vi "Test2_3a_ASIC_mezzanineNEW.vi"(4 "Voltages comprobation":dbl[](array[numeric])=[0.05, 0.1, 0.2, 0.3, 0.4, 0.5, 0.6, 0.7, 0.8, 1.0], 6 "IB_Clip":i32[](array[numeric])=[7, 15, 23, 31, 39, 47, 55, 63], 7 "Report Enable":bool, 8 "error in":errorcluster, 9 "Cycles Burst":i32=10000, 10 "Channels":i32[](array[numeric])=[0, 1, 2, 3, 4, 5, 6], 11 "Instrument VISA in":T1={"AWG VISA"="generadorpulsos", "Oscilloscope  VISA "="Oscilloscope", "Integration Board IP"="172.16.7.43", "connection ID"=refnum, "report out"=refnum, "report file path"=path "D:/CTA/Data_test/ASIC/chip_test"}) -> (0 "error out":errorcluster, 3 "Instrument VISA out":T1={"AWG VISA"="generadorpulsos", "Oscilloscope  VISA "="Oscilloscope", "Integration Board IP"="172.16.7.43", "connection ID"=refnum, "report out"=refnum, "report file path"=path "D:/CTA/Data_test/test3a"})   [LabVIEW 2009]
uses:
  <vilib>/Utility/NIReport.llb/NI_report.lvclass
  <vilib>/Utility/NIReport.llb/HTML/NI_HTML.lvclass
  <instrlib>/Agilent 8000 Series/Public/Configure/Configure Math (Binary Operation).vi
  <instrlib>/Agilent 8000 Series/Public/Data/Read (Multiple Waveforms).vi
  <instrlib>/Agilent 81150/Agilent 81150.lvlib
  L0_Asic/L0 Asic Test Folder v9/C/Program Files/National Instruments/LabVIEW 2012/instr.lib/Agilent 8000 Series/Agilent 8000 Series.lvlib
panel:
  in  "Selected Delay":i32=1
  in  "Atenuation":i32[](array[numeric])=[0, 4, 8, 12]
  in  "Generador enable?":bool=TRUE
  out "dt":dbl
  out "report file path":path=path "D:/CTA/Data_test/ASIC/chip_test"
  in  "Full waveform":bool
  out "Waveform Data":waveform(dbl)[](graph)
  out "x-y 4":u32=4294966934
  in  "y":dbl=250.0
  out "bucle":u16=32
  out "x-y 3":u32
  out "points quantity":dbl=10.0
  out "appended array":dbl[](array[numeric])=[9.99999e+37, 9.99999e+37, 9.99999e+37, 9.99999e+37, 0.028568, 0.000458, 2.716396e-09, 8.8051e-11, 1.4000634e-08, 8.5636e-11, 10.0]
  out "read buffer 3":string="V amptd(1),9.99999E+37,9.99999E+37,9.99999E+37,9.99999E+37,9.99999E+37,1.0E+01,+ width(1),9.99999E+37,9.99999E+37,9.99999E+37,9.99999E+37,9.99999E+37,9.99999E+37,V amptd(f2),2.861E-02,2.776E-02,2.904E-02,2.8568E-02,4.58E-04,1.0E+01,+ width(f2),2.81643E-09,2.57734E-09,2.81643E-09,2.716396E-09,8.8051E-11,1.0E+01,Time(1-f2),1.406011E-08,1.390256E-08,1.414073E-08,1.4000634E-08,8.5636E-11,1.0E+01\n"
  out "x-y":u32=372
  out "Numeric":i32=179238008
  in  "Att gain":u32=4095
  in  "Save NOW!":bool
  in  "End 2":bool
  out "Data output":dbl[][](array[numeric])=[[0.05, 0.0, 0.0, 0.0, 1.0, 9.99999e+37, 9.99999e+37, 9.99999e+37, 9.99999e+37, 9.99999e+37, 9.99999e+37, 9.99999e+37, 9.99999e+37, 9.99999e+37, 9.99999e+37, 11.0, 0.0336, 0.007807142857142857, 0.0], [0.05, 0.0, 0.0, 1.0, 1.0, 9.99999e+37, 9.99999e+37, 9.99999e+37, 9.99999e+37, 0.02322, 0.00108, 2.92182e-09, 1.2099e-10, 1.426508e-08, 1.0426e-10, 9.0, 0.0336, 0.007807142857142857, 1.0], [0.05, 0.0, 0.0, 2.0, 1.0, 9.99999e+37, 9.99999e+37, 9.99999e+37, 9.99999e+37, 0.027616, 0.00075, 2.762328e-09, 1.20518e-10, 1.396173e-08, 9.0461e-11, 10.0, 0.0336, 0.007807142857142857, 2.0], [0.05, 0.0, 0.0, 3.0, 1.0, 9.99999e+37, 9.99999e+37, 9.99999e+37, 9.99999e+37, 0.029619, 0.000653, 2.613329e-09, 9.9889e-11, 1.3763225e-08, 1.01914e-10, 10.0, 0.0336, 0.007807142857142857, 3.0], [0.05, 0.0, 0.0, 4.0, 1.0, 9.99999e+37, 9.99999e+37, 9.99999e+37, 9.99999e+37, 0.030934, 0.001529, 2.609376e-09, 5.0257e-11, 1.370877e-08, 6.3168e-11, 10.0, 0.0336, 0.007807142857142857, 4.0], [0.05, 0.0, 0.0, 5.0, 1.0, 9.99999e+37, 9.99999e+37, 9.99999e+37, 9.99999e+37, 0.031684, 0.000984, 2.569953e-09, 8.8766e-11, 1.3621526e-08, 6.259e-11, 10.0, 0.0336, 0.007807142857142857, 5.0], [0.05, 0.0, 0.0, 6.0, 1.0, 9.99999e+37, 9.99999e+37, 9.99999e+37, 9.99999e+37, 0.031778, 0.000782, 2.551811e-09, 9.6553e-11, 1.3593361e-08, 7.619e-11, 11.0, 0.0336, 0.007807142857142857, 6.0], [0.05, 1.0, 0.0, 0.0, 1.0, 9.99999e+37, 9.99999e+37, 9.99999e+37, 9.99999e+37, 9.99999e+37, 9.99999e+37, 9.99999e+37, 9.99999e+37, 1.011019e-08, 9.9856e-10, 10.0, 0.0336, 0.007807142857142857, 7.0], [0.05, 1.0, 0.0, 1.0, 1.0, 9.99999e+37, 9.99999e+37, 9.99999e+37, 9.99999e+37, 0.02143, 0.001274, 3.059757e-09, 1.55908e-10, 1.4327756e-08, 8.9144e-11, 10.0, 0.0336, 0.007807142857142857, 8.0], [0.05, 1.0, 0.0, 2.0, 1.0, 9.99999e+37, 9.99999e+37, 9.99999e+37, 9.99999e+37, 0.026315, 0.000821, 2.807153e-09, 5.1637e-11, 1.396698e-08, 1.01676e-10, 10.0, 0.0336, 0.007807142857142857, 9.0], [0.05, 1.0, 0.0, 3.0, 1.0, 9.99999e+37, 9.99999e+37, 9.99999e+37, 9.99999e+37, 0.028856, 0.001014, 2.729925e-09, 8.219e-11, 1.3780327e-08, 8.7828e-11, 10.0, 0.0336, 0.007807142857142857, 10.0], [0.05, 1.0, 0.0, 4.0, 1.0, 9.99999e+37, 9.99999e+37, 9.99999e+37, 9.99999e+37, 0.029136, 0.001454, 2.665592e-09, 8.3971e-11, 1.3697819e-08, 7.5969e-11, 10.0, 0.0336, 0.007807142857142857, 11.0], [0.05, 1.0, 0.0, 5.0, 1.0, 9.99999e+37, 9.99999e+37, 9.99999e+37, 9.99999e+37, 0.030325, 0.001136, 2.605316e-09, 7.6693e-11, 1.3613156e-08, 9.0082e-11, 10.0, 0.0336, 0.007807142857142857, 12.0], [0.05, 1.0, 0.0, 6.0, 1.0, 9.99999e+37, 9.99999e+37, 9.99999e+37, 9.99999e+37, 0.030542, 0.000695, 2.600691e-09, 7.2879e-11, 1.3579529e-08, 7.3212e-11, 11.0, 0.0336, 0.007807142857142857, 13.0], [0.05, 2.0, 0.0, 0.0, 1.0, 9.99999e+37, 9.99999e+37, 9.99999e+37, 9.99999e+37, 9.99999e+37, 9.99999e+37, 9.99999e+37, 9.99999e+37, 9.99999e+37, 9.99999e+37, 10.0, 0.0336, 0.007807142857142857, 14.0], [0.05, 2.0, 0.0, 1.0, 1.0, 9.99999e+37, 9.99999e+37, 9.99999e+37, 9.99999e+37, 0.019386, 0.000608, 3.093134e-09, 1.37969e-10, 1.428753e-08, 1.14612e-10, 10.0, 0.0336, 0.007807142857142857, 15.0], [0.05, 2.0, 0.0, 2.0, 1.0, 9.99999e+37, 9.99999e+37, 9.99999e+37, 9.99999e+37, 0.024483, 0.000731, 2.928339e-09, 1.06101e-10, 1.4002377e-08, 6.2052e-11, 10.0, 0.0336, 0.007807142857142857, 16.0], [0.05, 2.0, 0.0, 3.0, 1.0, 9.99999e+37, 9.99999e+37, 9.99999e+37, 9.99999e+37, 0.027198, 0.001369, 2.781238e-09, 5.6434e-11, 1.386892e-08, 9.0615e-11, 11.0, 0.0336, 0.007807142857142857, 17.0], [0.05, 2.0, 0.0, 4.0, 1.0, 9.99999e+37, 9.99999e+37, 9.99999e+37, 9.99999e+37, 0.029441, 0.001219, 2.623158e-09, 6.7678e-11, 1.3704754e-08, 8.6571e-11, 11.0, 0.0336, 0.007807142857142857, 18.0], [0.05, 2.0, 0.0, 5.0, 1.0, 9.99999e+37, 9.99999e+37, 9.99999e+37, 9.99999e+37, 0.030537, 0.000977, 2.611114e-09, 5.8592e-11, 1.365028e-08, 5.1809e-11, 10.0, 0.0336, 0.007807142857142857, 19.0], [0.05, 2.0, 0.0, 6.0, 1.0, 9.99999e+37, 9.99999e+37, 9.99999e+37, 9.99999e+37, 0.031627, 0.000829, 2.563156e-09, 7.6101e-11, 1.3573521e-08, 7.8038e-11, 11.0, 0.0336, 0.007807142857142857, 20.0], [0.05, 3.0, 0.0, 0.0, 1.0, 9.99999e+37, 9.99999e+37, 9.99999e+37, 9.99999e+37, 9.99999e+37, 9.99999e+37, 9.99999e+37, 9.99999e+37, 9.99999e+37, 9.99999e+37, 10.0, 0.0336, 0.007807142857142857, 21.0], [0.05, 3.0, 0.0, 1.0, 1.0, 9.99999e+37, 9.99999e+37, 9.99999e+37, 9.99999e+37, 0.023426, 0.000976, 2.943703e-09, 1.24879e-10, 1.4377233e-08, 6.3364e-11, 10.0, 0.0336, 0.007807142857142857, 22.0], [0.05, 3.0, 0.0, 2.0, 1.0, 9.99999e+37, 9.99999e+37, 9.99999e+37, 9.99999e+37, 0.027462, 0.001241, 2.749469e-09, 8.035e-11, 1.407543e-08, 9.5871e-11, 10.0, 0.0336, 0.007807142857142857, 23.0], [0.05, 3.0, 0.0, 3.0, 1.0, 9.99999e+37, 9.99999e+37, 9.99999e+37, 9.99999e+37, 0.030115, 0.000527, 2.608621e-09, 5.3293e-11, 1.3888327e-08, 4.0853e-11, 10.0, 0.0336, 0.007807142857142857, 24.0], [0.05, 3.0, 0.0, 4.0, 1.0, 9.99999e+37, 9.99999e+37, 9.99999e+37, 9.99999e+37, 0.030314, 0.000803, 2.543724e-09, 8.472e-11, 1.3780628e-08, 6.8952e-11, 11.0, 0.0336, 0.007807142857142857, 25.0], [0.05, 3.0, 0.0, 5.0, 1.0, 9.99999e+37, 9.99999e+37, 9.99999e+37, 9.99999e+37, 0.030543, 0.000778, 2.505925e-09, 4.3746e-11, 1.3739439e-08, 4.7108e-11, 10.0, 0.0336, 0.007807142857142857, 26.0], [0.05, 3.0, 0.0, 6.0, 1.0, 9.99999e+37, 9.99999e+37, 9.99999e+37, 9.99999e+37, 0.03222, 0.00104, 2.47222e-09, 7.807e-11, 1.366951e-08, 7.53e-11, 9.0, 0.0336, 0.007807142857142857, 27.0], [0.05, 4.0, 0.0, 0.0, 1.0, 9.99999e+37, 9.99999e+37, 9.99999e+37, 9.99999e+37, 9.99999e+37, 9.99999e+37, 1.195182e-08, 8.02096e-09, 3.628837e-09, 9.761988e-09, 10.0, 0.0336, 0.007807142857142857, 28.0], [0.05, 4.0, 0.0, 1.0, 1.0, 9.99999e+37, 9.99999e+37, 9.99999e+37, 9.99999e+37, 0.021167, 0.000405, 3.005073e-09, 1.20406e-10, 1.4438271e-08, 1.02183e-10, 10.0, 0.0336, 0.007807142857142857, 29.0], [0.05, 4.0, 0.0, 2.0, 1.0, 9.99999e+37, 9.99999e+37, 9.99999e+37, 9.99999e+37, 0.025505, 0.00093, 2.873754e-09, 5.6494e-11, 1.4181106e-08, 7.6256e-11, 11.0, 0.0336, 0.007807142857142857, 30.0], [0.05, 4.0, 0.0, 3.0, 1.0, 9.99999e+37, 9.99999e+37, 9.99999e+37, 9.99999e+37, 0.028568, 0.000458, 2.716396e-09, 8.8051e-11, 1.4000634e-08, 8.5636e-11, 10.0, 0.0336, 0.007807142857142857, 31.0]]
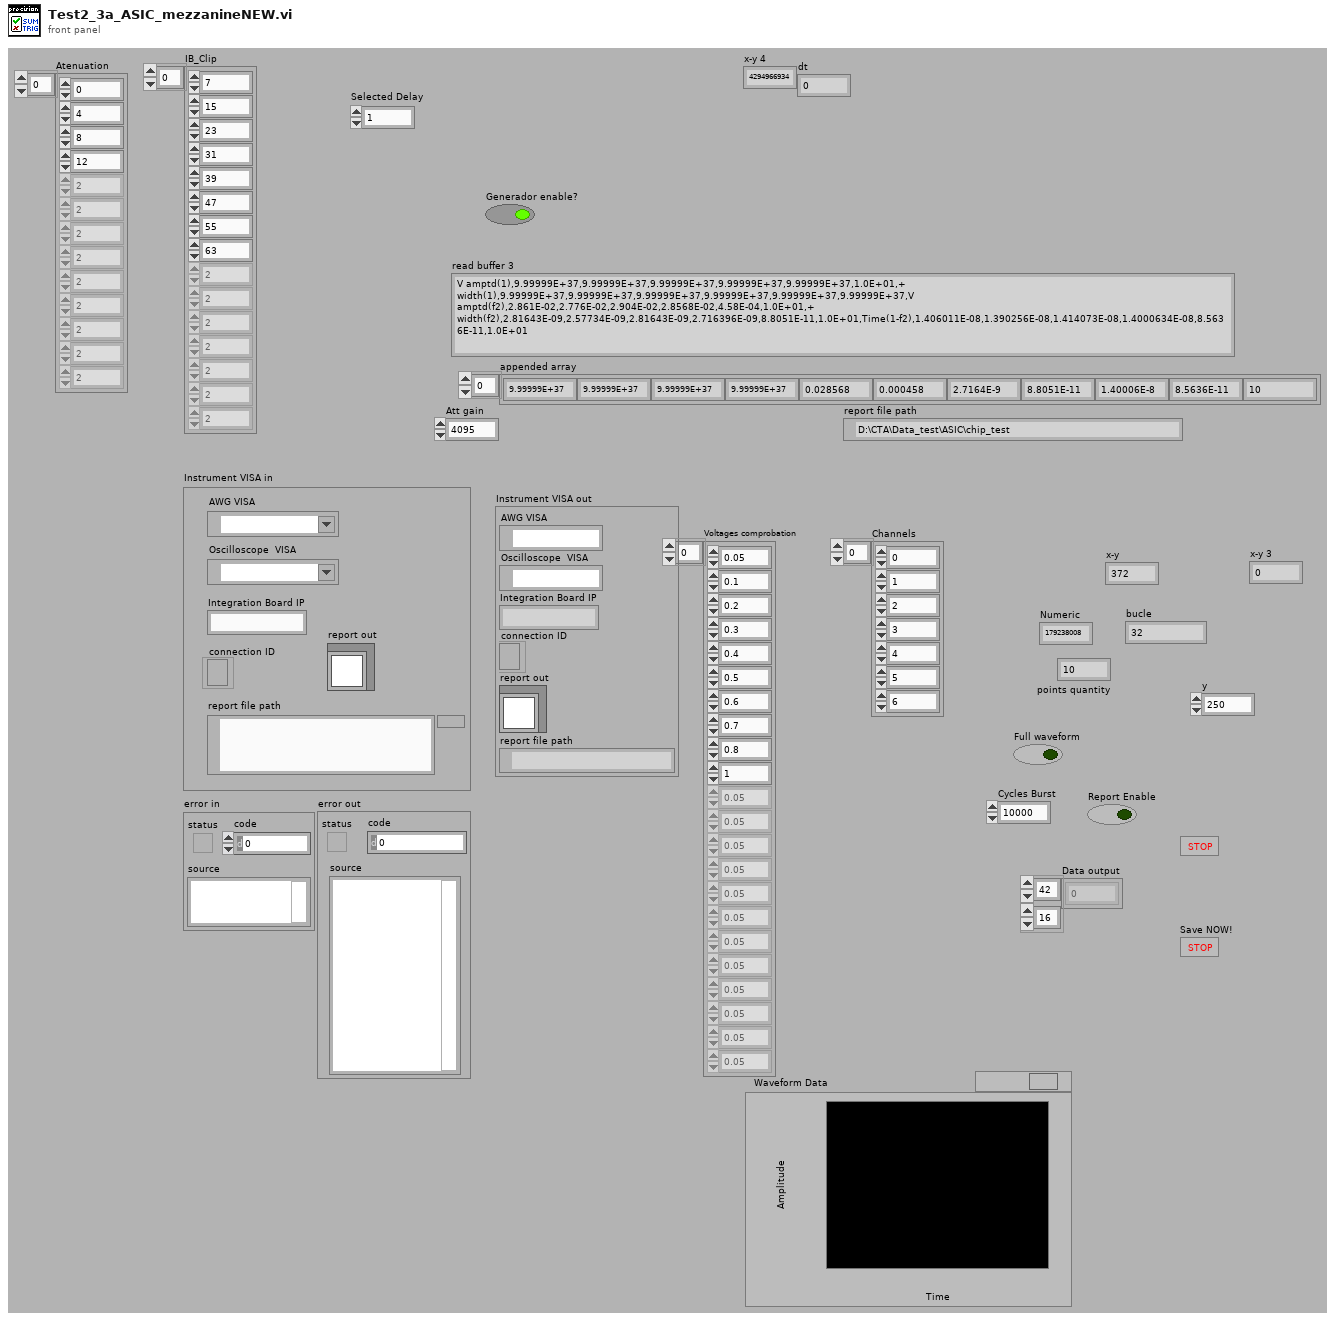
[diagram p1: front panel]
types:
  T1 = cluster{"AWG VISA":refnum<visa-resource-name>, "Oscilloscope  VISA ":refnum<visa-resource-name>, "Integration Board IP":string, "connection ID":refnum<k5>, "report out":refnum<class "NI_report.lvclass">, "report file path":path}
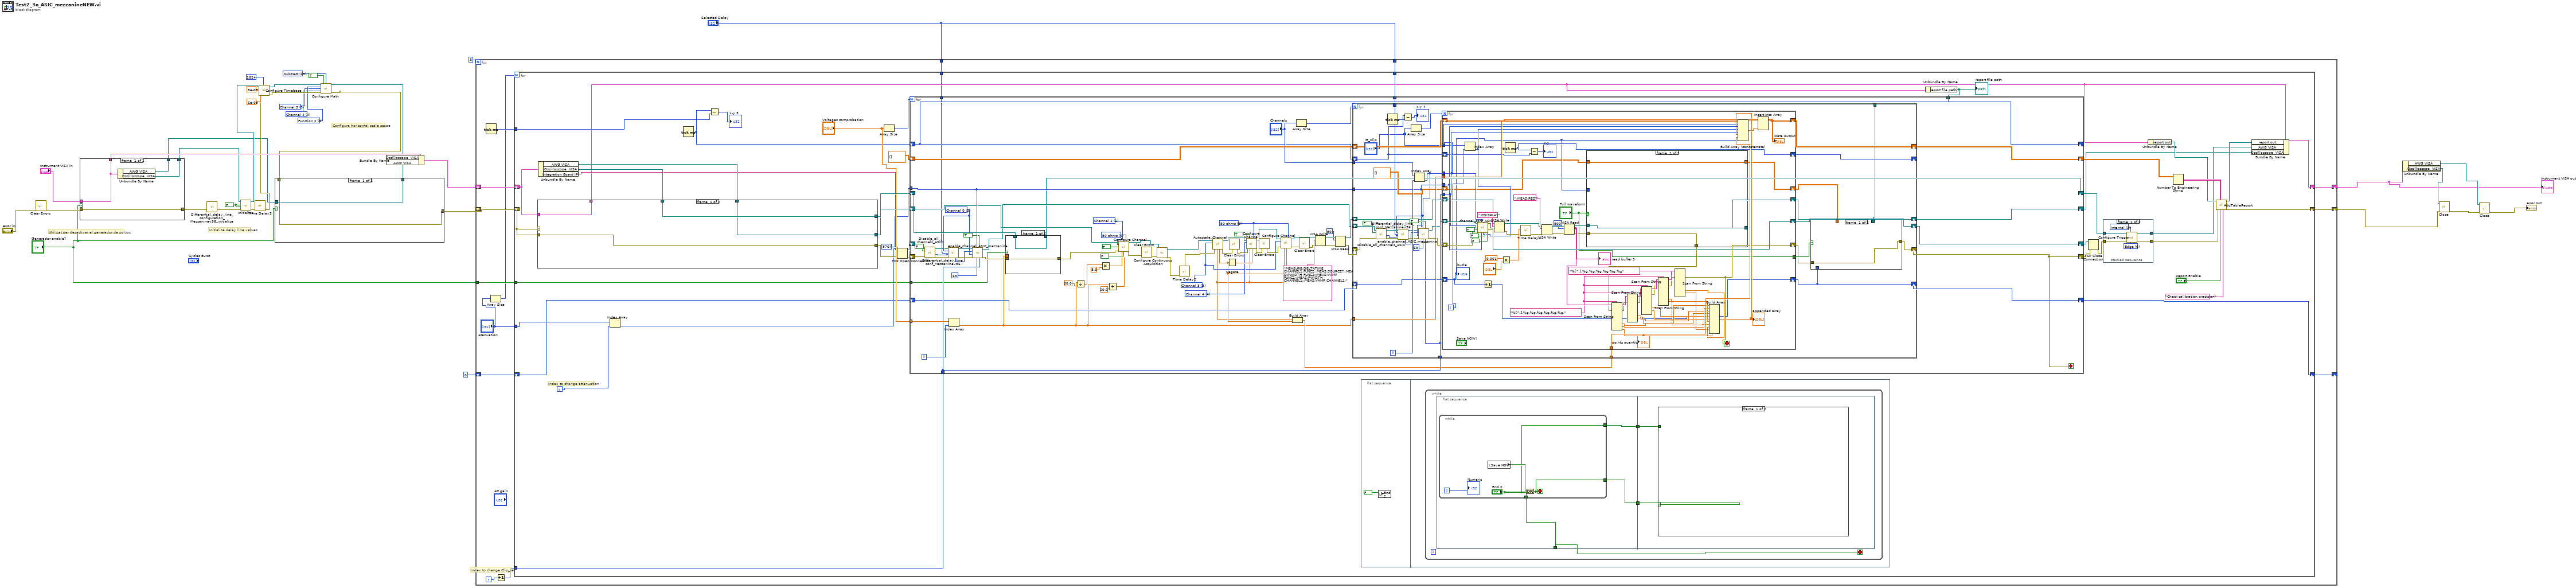
[diagram p0: block diagram]
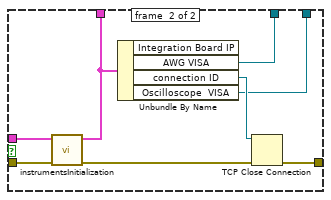
[diagram p2: hidden frame]
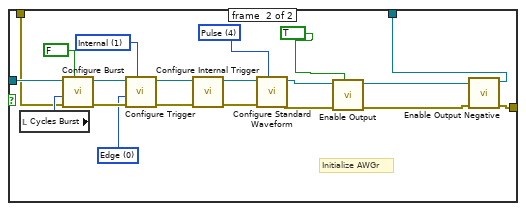
[diagram p3: hidden frame]
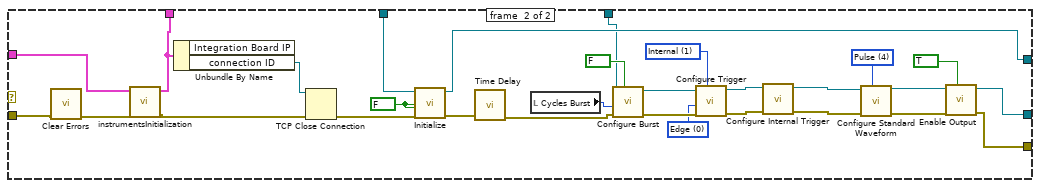
[diagram p4: hidden frame]
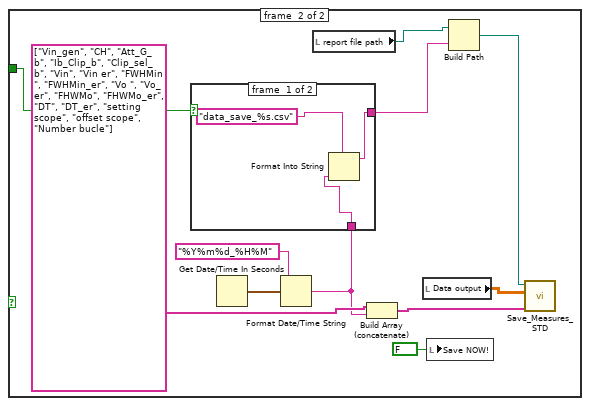
[diagram p5: hidden frame]
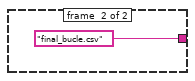
[diagram p6: hidden frame]
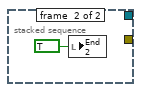
[diagram p7: hidden frame]
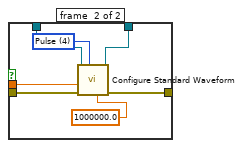
[diagram p8: hidden frame]
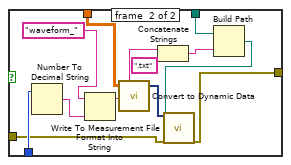
[diagram p9: hidden frame]
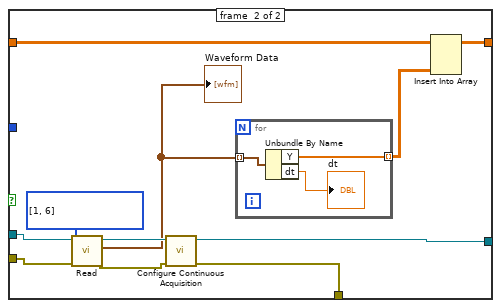
[diagram p10: hidden frame]
diagram:
  w25 = u16 6 items=["Function 1"=5, "Function 2"=6, "Function 3"=7, "Function 4"=8] ("Math Channel (5: Function 1)")
  w29 = u16 15 items=["Add"=12, "Divide"=13, "Multiply"=14, "Subtract"=15, "Common Mode"=16, "Versus"=17] ("Math Operation (12: Add)")
  w24 = 3 items=["Channel 1"=1, "Channel 2"=2, "Channel 3"=3, "Channel 4"=4] ("Channel (1: Channel 1)")
  w23 = 4 items=["Channel 1"=1, "Channel 2"=2, "Channel 3"=3, "Channel 4"=4] ("Channel (1: Channel 1)")
  w37 = FALSE ("ID Query (True)")
  # "Configure horizontal scale scope"
  # "Initialize delay line values"
  # "Utilitzat per desactivar el generador de polsos"
  # "Index to change Clip_sel"
  n1 = call <vilib>:"Clear Errors.vi"("error in (no error)"="error in") -> ("error out"=w35:errorcluster)  [unwired: 6 in]
  n2 = case shown="True" "Generador enable?" {
    tunnel: w35 -> [w41 w49]
    tunnel: "Instrument VISA in" -> [w38 w48]
    tunnel: [w38 w47] -> w32
    tunnel: [w41 w42] -> w5
    tunnel: [w40 w44] -> w4
    tunnel: [w39 w45] -> w3
    frame #0 {
      n3 = Unbundle By Name(w38) -> ("AWG VISA"=w40:refnum<visa-resource-name>, "Oscilloscope  VISA"=w39:refnum<visa-resource-name>)
    }
    frame #1 {
      n4 = call "instrumentsInitialization.vi"("error in"=w49, "Instrument VISA in"=w48) -> ("error out"=w43:errorcluster, "Instrument VISA out"=w47:T1)  [unwired: 8 in]
      n5 = Unbundle By Name(w47) -> ("AWG VISA"=w44:refnum<visa-resource-name>, "connection ID"=w46:refnum<k5>, "Oscilloscope  VISA"=w45:refnum<visa-resource-name>)  [unwired: 1 out]
      n6 = TCP Close Connection(connection ID=w46, error in (no error)=w43) -> (error out=w42:errorcluster)  [unwired: 1 in, 1 out]
    }
  }
  n7 = call "Differential_delay_line_configuration_Mezzaninev56_initialize.vi"("error in (no error)"=w5) -> ("error out 2"=w6:errorcluster)  [unwired: 1 in]
  n8 = call "Initialize.vi"("error in (no error)"=w6, "Reset (True)"=w37, "ID Query (True)"=w37, "VISA resource name"=w3) -> ("error out"=w36:errorcluster, "VISA resource name out"=w22:refnum<visa-resource-name>)  [unwired: 6 in]
  n9 = call "Time Delay3"("error in (no error)"=w36) -> ("error out"=w21:errorcluster)  [unwired: 10 in]
  n10 = call "Configure Timebase.vi"("Record Length (1000)"=1024, "error in (no error)"=w21, "Position (0.0 s)"=6e-09, "Timebase (0.005 s)"=5e-08, "VISA resource name"=w22) -> ("error out"=w26:errorcluster, "VISA resource name out"=w27:refnum<visa-resource-name>)  [unwired: 5 in]
  n11 = call-poly <instrlib>:"Configure Math.vi"("VISA resource name"=w27, "Enable Math Channel (T:Enable)"=TRUE, "Math Operation (12: Add)"=w29, "Math Channel (5: Function 1)"=w25, "Math Operand (1: Channel 1)"=w24, "Math Operand (2: Channel 2)"=w23, "error in (no error)"=w26) -> ("VISA resource name out"=w10:refnum<visa-resource-name>, "error out"=w11:errorcluster)  [unwired: 7 in]
  n12 = case shown="True" "Generador enable?" {
    tunnel: w4 -> [w50 w60]
    tunnel: w11 -> [w51 w56]
    tunnel: [w51 w54] -> w8
    tunnel: [w50 w52] -> w7
    frame #0 {
    }
    frame #1 {
      w65 = u16 1 items=["Immediate", "Internal", "External", "Software Trigger Function"] ("Trigger Source (0: Immediate)")
      w66 = u16 0 items=["Edge", "Level"] ("Trigger Mode (0: Edge)")
      w70 = u16 4 items=["Sine", "Square", "Ramp Up", "Ramp Down", "Pulse", "Noise", "DC"] ("Waveform (0: Sine)")
      # "Initialize AWGr"
      n13 = local read "Cycles Burst"() -> (w69:i32)
      n14 = call <instrlib>:"Configure Burst.vi"("Enable Burst (F: Disable)"=FALSE, "error in (no error)"=w56, "Burst Count (2)"=w69, "VISA resource name"=w60) -> ("error out"=w68:errorcluster, "VISA resource name out"=w67:refnum<visa-resource-name>)  [unwired: 6 in]
      n15 = call <instrlib>:"Configure Trigger.vi"("Trigger Source (0: Immediate)"=w65, "error in (no error)"=w68, "Trigger Mode (0: Edge)"=w66, "VISA resource name"=w67) -> ("error out"=w64:errorcluster, "VISA resource name out"=w63:refnum<visa-resource-name>)  [unwired: 6 in]
      n16 = call <instrlib>:"Configure Internal Trigger.vi"("error in (no error)"=w64, "VISA resource name"=w63) -> ("error out"=w61:errorcluster, "VISA resource name out"=w62:refnum<visa-resource-name>)  [unwired: 8 in]
      n17 = call <instrlib>:"Configure Standard Waveform.vi"("Waveform (0: Sine)"=w70, "error in (no error)"=w61, "VISA resource name"=w62) -> ("error out"=w59:errorcluster, "VISA resource name out"=w58:refnum<visa-resource-name>)  [unwired: 7 in]
      n18 = call <instrlib>:"Enable Output.vi"("Enable Output (T: Enable)"=TRUE, "error in (no error)"=w59, "VISA resource name"=w58) -> ("error out"=w55:errorcluster, "VISA resource name out"=w53:refnum<visa-resource-name>)  [unwired: 7 in]
      n19 = call <instrlib>:"Enable Output Negative.vi"("error in (no error)"=w55, "VISA resource name"=w53) -> ("error out"=w54:errorcluster, "VISA resource name out"=w52:refnum<visa-resource-name>)  [unwired: 8 in]
    }
  }
  n20 = Bundle By Name(cluster=w32, "Oscilloscope  VISA"=w10, "AWG VISA"=w7) -> (w13:T1)
  n21 = for {
    N: 3 -> [_]
    shift-right: [w85] -> w16
    shift-left: w8 -> [w81]
    shift-right: [w84] -> w14
    shift-left: w13 -> [w80]
    shift-right: [w77] -> _
    shift-left: u16 0 ("remote port or service name") -> [w78]
    tunnel: "Generador enable?" -> [w76]
    tunnel: "Selected Delay" -> [w73]
    tunnel: "Selected Delay" -> [w72]
    i -> [w82]
    n22 = Tick Count (ms)() -> (millisecond timer value=w79:u32)
    n23 = Array Size(array="Atenuation") -> (size(s)=w74:i32)
    n24 = Increment(x=w82) -> (x+1=w83:i32)
    n25 = for {
      N: w74 -> [_]
      shift-right: [w119] -> w85
      shift-left: w81 -> [w113]
      shift-right: [w117] -> w84
      shift-left: w80 -> [w118]
      tunnel: w83 -> [w92]
      tunnel: w79 -> [w99]
      shift-right: [w97] -> w77
      shift-left: w78 -> [w98]
      tunnel: w76 -> [w91]
      tunnel: "Atenuation" -> [w89]
      tunnel: w73 -> [w87]
      tunnel: w72 -> [w86]
      i -> [w88]
      # "Index to change attenuation"
      n26 = Unbundle By Name(w118) -> ("AWG VISA"=w112:refnum<visa-resource-name>, "Oscilloscope  VISA"=w115:refnum<visa-resource-name>, "Integration Board IP"=w108:string)
      n27 = case shown="Error" w113 {
        tunnel: w118 -> [w132 w161]
        tunnel: w113 -> [w131 w155]
        tunnel: [w132 w160] -> w94
        tunnel: [w131 w137] -> w107
        tunnel: w115 -> [w130 w159]
        tunnel: [w130 w158] -> w114
        tunnel: w112 -> [w129 w139]
        tunnel: [w129 w138] -> w111
        frame #0 {
        }
        frame #1 {
          w144 = u16 1 items=["Immediate", "Internal", "External", "Software Trigger Function"] ("Trigger Source (0: Immediate)")
          w145 = u16 0 items=["Edge", "Level"] ("Trigger Mode (0: Edge)")
          w152 = u16 4 items=["Sine", "Square", "Ramp Up", "Ramp Down", "Pulse", "Noise", "DC"] ("Waveform (0: Sine)")
          w157 = FALSE ("ID Query (True)")
          n28 = call <vilib>:"Clear Errors.vi"("error in (no error)"=w155) -> ("error out"=w154:errorcluster)  [unwired: 6 in]
          n29 = call "instrumentsInitialization.vi"("error in"=w154, "Instrument VISA in"=w161) -> ("error out"=w134:errorcluster, "Instrument VISA out"=w160:T1)  [unwired: 8 in]
          n30 = Unbundle By Name(w160) -> ("connection ID"=w135:refnum<k5>)  [unwired: 1 out]
          n31 = TCP Close Connection(connection ID=w135, error in (no error)=w134) -> (error out=w133:errorcluster)  [unwired: 1 in, 1 out]
          n32 = call "Initialize.vi"("error in (no error)"=w133, "Reset (True)"=w157, "ID Query (True)"=w157, "VISA resource name"=w159) -> ("error out"=w156:errorcluster, "VISA resource name out"=w158:refnum<visa-resource-name>)  [unwired: 6 in]
          n33 = call "Time Delay"("error in (no error)"=w156) -> ("error out"=w136:errorcluster)  [unwired: 10 in]
          n34 = local read "Cycles Burst"() -> (w148:i32)
          n35 = call <instrlib>:"Configure Burst.vi"("Enable Burst (F: Disable)"=FALSE, "error in (no error)"=w136, "Burst Count (2)"=w148, "VISA resource name"=w139) -> ("error out"=w147:errorcluster, "VISA resource name out"=w146:refnum<visa-resource-name>)  [unwired: 6 in]
          n36 = call <instrlib>:"Configure Trigger.vi"("Trigger Source (0: Immediate)"=w144, "error in (no error)"=w147, "Trigger Mode (0: Edge)"=w145, "VISA resource name"=w146) -> ("error out"=w143:errorcluster, "VISA resource name out"=w142:refnum<visa-resource-name>)  [unwired: 6 in]
          n37 = call <instrlib>:"Configure Internal Trigger.vi"("error in (no error)"=w143, "VISA resource name"=w142) -> ("error out"=w140:errorcluster, "VISA resource name out"=w141:refnum<visa-resource-name>)  [unwired: 8 in]
          n38 = call <instrlib>:"Configure Standard Waveform.vi"("Waveform (0: Sine)"=w152, "error in (no error)"=w140, "VISA resource name"=w141) -> ("error out"=w151:errorcluster, "VISA resource name out"=w150:refnum<visa-resource-name>)  [unwired: 7 in]
          n39 = call <instrlib>:"Enable Output.vi"("Enable Output (T: Enable)"=TRUE, "error in (no error)"=w151, "VISA resource name"=w150) -> ("error out"=w137:errorcluster, "VISA resource name out"=w138:refnum<visa-resource-name>)  [unwired: 7 in]
        }
      }
      n40 = Index Array(array=w89, index=w88) -> (element=w90:i32)
      n41 = Tick Count (ms)() -> (millisecond timer value=w100:u32)
      n42 = Subtract(x=w100, y=w99) -> (x-y=→"x-y 3":u32)
      n43 = Array Size(array="Voltages comprobation") -> (size(s)=w120:i32)
      n44 = TCP Open Connection(address=w108, remote port or service name=u16 9764, error in (no error)=w107) -> (connection ID=w102:refnum<k5>, error out=w106:errorcluster)  [unwired: 2 in]
      n45 = flat-sequence {
        frame #0 {
          n46 = local write "End 2"(FALSE ("End")) -> ()
        }
        frame #1 {
          n47 = while {
            stop <- w163 stop-if-true
            n48 = flat-sequence {
              tunnel: [w168] -> w165
              tunnel: [w167] -> w164
              tunnel: [w166] -> w163
              tunnel: w165 -> [w174]
              tunnel: w164 -> [w173]
              frame #0 {
                n49 = while {
                  tunnel: [w171] -> w168
                  tunnel: ["End 2"] -> w167
                  tunnel: ["End 2"] -> w166
                  i -> [w170]
                  stop <- w171 stop-if-true
                  n50 = local read "Save NOW!"() -> (w172:bool)
                  n51 = Or(x=w172, y="End 2") -> (x .or. y?=w171:bool)
                  "Numeric" <- w170
                }
              }
              frame #1 {
                n52 = case shown="True" w174 {
                  tunnel: w173 -> [_ w182]
                  frame #0 {
                  }
                  frame #1 {
                    n53 = Get Date/Time In Seconds() -> (seconds since 1Jan1904=w178:timestamp)
                    n54 = Format Date/Time String(time format string (%c)="%Y%m%d_%H%M", seconds (now)=w178) -> (date/time string=w176:string)  [unwired: 1 in]
                    n55 = case shown="False" w182 {
                      tunnel: [w187 "final_bucle.csv" ("format string")] -> w181
                      tunnel: w176 -> [w186 _]
                      frame #0 {
                        n56 = Format Into String(format string="data_save_%s.csv", w186) -> (resulting string=w187:string)  [unwired: 2 in, 1 out]
                      }
                      frame #1 {
                      }
                    }
                    n57 = local read "report file path"() -> (w175:path)
                    n58 = Build Array (concatenate)(string[] ["Vin_gen", "CH", "Att_G_b", "Ib_Clip_b", "Clip_sel_b", "Vin", "Vin er", "FWHMin ", "FWHMin_er", "Vo ", "Vo_er", "FHWMo", "FHWMo_er", "DT", "DT_er", "setting scope", "offset scope", "Number bucle"] ("appended array"), w176) -> (w179:string[])
                    n59 = local read "Data output"() -> (w184:dbl[][])
                    n60 = local write "Save NOW!"(FALSE ("Save NOW!")) -> ()
                    n61 = Build Path(base path=w175, name or relative path=w181) -> (appended path=w185:path)
                    n62 = call "Save_Measures_STD.vi"("appended array"=w179, "Data in"=w184, "file path (dialog if empty)"=w185) -> ()  [unwired: 9 in]
                  }
                }
              }
            }
          }
        }
      }
      n63 = Unbundle By Name(w94) -> ("report file path"=w93:path)
      "report file path" <- w93
      n64 = for {
        N: w120 -> [_]
        shift-right: [w210] -> w104
        shift-left: w106 -> [w242]
        shift-right: [w265] -> w124
        shift-left: dbl[][] [] -> [w266]
        tunnel: "Voltages comprobation" -> [w264]
        shift-right: [w230] -> w116
        shift-left: w111 -> [w272]
        shift-right: [w258] -> w95
        shift-left: w114 -> [w247]
        tunnel: w90 -> [w256]
        tunnel: w92 -> [w253]
        shift-right: [w241] -> w103
        shift-left: w102 -> [w240]
        shift-right: [w213] -> _
        shift-left: w100 -> [w213]
        shift-right: [w212] -> w97
        shift-left: w98 -> [w226]
        tunnel: w93 -> [w211]
        tunnel: w91 -> [w199]
        tunnel: w87 -> [w198]
        tunnel: w86 -> [w197]
        i -> [w271]
        stop <- w210 stop-if-true
        w219 = 3 items=["Channel 1"=1, "Channel 2"=2, "Channel 3"=3, "Channel 4"=4] ("Channel (1: Channel 1)")
        w243 = 4 items=["Channel 1"=1, "Channel 2"=2, "Channel 3"=3, "Channel 4"=4] ("Channel (1: Channel 1)")
        w220 = u32 0 items=["50 ohms", "1 Mohms"] ("Input Impedance (1: 1 Mohms)")
        w205 = u16 0 items=["Channel 0", "Channel 1", "Channel 2", "Channel 3", "Channel 4", "Channel 5", "Channel 6"] ("Channel")
        w268 = u32 0 items=["50 ohms", "1 Mohms"] ("Input Impedance (1: 1 Mohms)")
        w270 = 1 items=["Channel 1"=1, "Channel 2"=2, "Channel 3"=3, "Channel 4"=4] ("Channel (1: Channel 1)")
        n65 = call "Disable_all_channels_ASIC.vi"("error in"=w242, "Clip_en_b"=FALSE, "connection ID"=w240) -> ("error out"=w206:errorcluster, "id_out"=w209:i32, "connection ID out"=w203:refnum<k5>)  [unwired: 6 in]
        n66 = call "Differential_delay_line_conf_Mezzaninev56.vi"("connection ID"=w203, "channel"=w205, "Delay value"=w198, "Id in"=w209, "error in (no error)"=w206) -> ("connection ID out"=w204:refnum<k5>, "Id out"=w208:i32, "error out 2"=w207:errorcluster)  [unwired: 3 in, 5 out]
        n67 = Index Array(array=w264, index=w271) -> (element=w202:dbl)
        n68 = call "enable_channel_ASIC_mezzanine.vi"("Clip_sel_b"=w253, "maj/sum"=TRUE, "Ib_clipVb"=u32 63, "Att gain"=w256, "error in"=w207, "Channel"=w205, "id_in"=w208, "connection ID"=w204) -> ("error out"=w257:errorcluster, "connection ID out"=w232:refnum<k5>)  [unwired: 1 in, 1 out]
        n69 = case shown="True" w199 {
          tunnel: w272 -> [w273 w279]
          tunnel: w257 -> [w274 w278]
          tunnel: [w274 w277] -> w248
          tunnel: [w273 w276] -> w230
          tunnel: w202 -> [_ w275]
          frame #0 {
          }
          frame #1 {
            w280 = u16 4 items=["Sine", "Square", "Ramp Up", "Ramp Down", "Pulse", "Noise", "DC"] ("Waveform (0: Sine)")
            n70 = call <instrlib>:"Configure Standard Waveform.vi"("Frequency (1000.0 Hz)"=1000000.0, "Waveform (0: Sine)"=w280, "error in (no error)"=w278, "Amplitude (1.0 Vpp)"=w275, "VISA resource name"=w279) -> ("error out"=w277:errorcluster, "VISA resource name out"=w276:refnum<visa-resource-name>)  [unwired: 5 in]
          }
        }
        n71 = Divide(x=w202, y=30.0) -> (x/y=w200:dbl)
        n72 = Multiply(x=w200, y=8.0) -> (x*y=w251:dbl)
        n73 = Divide(x=w202, y=20.0) -> (x/y=w255:dbl)
        n74 = call "Configure Channel.vi"("VISA resource name"=w247, "Enable Channel (Enable)"=TRUE, "BW Limit 20MHz (Disable)"=FALSE, "Input Impedance (1: 1 Mohms)"=w268, "Channel (1: Channel 1)"=w270, "error in (no error)"=w248, "Vertical Range (2.0 V)"=w251, "Vertical Offset (0.0 V)"=w255) -> ("VISA resource name out"=w246:refnum<visa-resource-name>, "error out"=w245:errorcluster)  [unwired: 6 in]
        n75 = call <vilib>:"Clear Errors.vi"("error in (no error)"=w245) -> ("error out"=w244:errorcluster)  [unwired: 6 in]
        n76 = call "Configure Continuous Acquisition.vi"("error in (no error)"=w244, "VISA resource name"=w246) -> ("error out"=w254:errorcluster, "VISA resource name out"=w238:refnum<visa-resource-name>)  [unwired: 8 in]
        n77 = call "Time Delay2"("error in (no error)"=w254) -> ("error out"=w239:errorcluster)  [unwired: 10 in]
        n78 = call "Autoscale_Channel.vi"("error in"=w239, "Channel"=w219, "VISA resource name"=w238) -> ("error out"=w259:errorcluster, "VISA resource name out"=w262:refnum<visa-resource-name>, "Offset"=w218:dbl, "VerticalRange"=w217:dbl)  [unwired: 5 in]
        n79 = Negate(x=w218) -> (-x=w249:dbl)
        n80 = call <vilib>:"Clear Errors.vi"("error in (no error)"=w259) -> ("error out"=w260:errorcluster)  [unwired: 6 in]
        n81 = call "Configure Channel.vi"("VISA resource name"=w262, "Enable Channel (Enable)"=TRUE, "Input Impedance (1: 1 Mohms)"=w220, "Channel (1: Channel 1)"=w243, "error in (no error)"=w260, "Vertical Range (2.0 V)"=w217, "Vertical Offset (0.0 V)"=w249) -> ("VISA resource name out"=w222:refnum<visa-resource-name>, "error out"=w261:errorcluster)  [unwired: 7 in]
        n82 = call <vilib>:"Clear Errors.vi"("error in (no error)"=w261) -> ("error out"=w224:errorcluster)  [unwired: 6 in]
        n83 = call "Configure Channel.vi"("VISA resource name"=w222, "Input Impedance (1: 1 Mohms)"=w220, "Channel (1: Channel 1)"=w219, "error in (no error)"=w224, "Vertical Range (2.0 V)"=w217, "Vertical Offset (0.0 V)"=w218) -> ("VISA resource name out"=w221:refnum<visa-resource-name>, "error out"=w225:errorcluster)  [unwired: 8 in]
        n84 = Build Array(w217, w218) -> (w250:dbl[])
        n85 = Array Size(array="Channels") -> (size(s)=w231:i32)
        n86 = call <vilib>:"Clear Errors.vi"("error in (no error)"=w225) -> ("error out"=w223:errorcluster)  [unwired: 6 in]
        n87 = VISA Write(VISA resource name=w221, write buffer="MEASURE:DELTATIME CHANNEL1,FUNC2;:MEAS:SOURCE?;:MEAS:PWIDTH FUNC2;:MEAS:VAMP FUNC2;:MEAS:PWIDTH CHANNEL1;:MEAS:VAMP CHANNEL1;", error in (no error)=w223) -> (VISA resource name out=w237:refnum<visa-resource-name>, error out=w236:errorcluster)  [unwired: 1 out]
        n88 = VISA Read(VISA resource name=w237, byte count=u32 50, error in (no error)=w236) -> (VISA resource name out=w233:refnum<visa-resource-name>, error out=w234:errorcluster)  [unwired: 2 out]
        n89 = for {
          N: w231 -> [_]
          tunnel: w256 -> [w285]
          tunnel: w253 -> [w305]
          tunnel: w202 -> [w318]
          tunnel: w250 -> [w317]
          shift-right: [w320] -> w265
          shift-left: w266 -> [w321]
          shift-right: [w319] -> w258
          shift-left: w233 -> [w315]
          shift-right: [w316] -> w241
          shift-left: w232 -> [w309]
          shift-right: [w297] -> w210
          shift-left: w234 -> [w311]
          tunnel: "Channels" -> [w314]
          shift-right: [w293] -> w212
          shift-left: w226 -> [w312]
          shift-right: [w299] -> _
          shift-left: w213 -> [w300]
          tunnel: w211 -> [w295]
          tunnel: w197 -> [w282]
          i -> [w313]
          n90 = call "Disable_all_channels_ASIC.vi"("error in"=w311, "Clip_en_b"=FALSE, "connection ID"=w309) -> ("error out"=w289:errorcluster, "id_out"=w286:i32, "connection ID out"=w291:refnum<k5>)  [unwired: 6 in]
          n91 = Tick Count (ms)() -> (millisecond timer value=w301:u32)
          n92 = Subtract(x=w300, y=w301) -> (x-y=→"x-y 4":u32)
          n93 = Array Size(array="IB_Clip") -> (size(s)=w303:i32)
          n94 = Index Array(array=w314, index=w313) -> (element=w284:i32)
          n95 = call "Differential_delay_line_conf_Mezzaninev56.vi"("connection ID"=w291, "channel"=w284, "Delay value"=w282, "Id in"=w286, "error in (no error)"=w289) -> ("connection ID out"=w290:refnum<k5>, "Id out"=w287:i32, "error out 2"=w288:errorcluster)  [unwired: 3 in, 5 out]
          n96 = call "enable_channel_ASIC_mezzanine.vi"("Clip_sel_b"=w305, "maj/sum"=TRUE, "Ib_clipVb"=u32 63, "Att gain"=w285, "error in"=w288, "Channel"=w284, "id_in"=w287, "connection ID"=w290) -> ("error out"=w310:errorcluster, "connection ID out"=w308:refnum<k5>)  [unwired: 1 in, 1 out]
          n97 = for {
            N: w303 -> [_]
            shift-right: [w338] -> w296
            shift-left: w310 -> [w365]
            tunnel: w318 -> [w400]
            shift-right: [w378] -> w320
            shift-left: w321 -> [w398]
            tunnel: w285 -> [w395]
            shift-right: [w341] -> w319
            shift-left: w315 -> [w367]
            tunnel: w305 -> [w394]
            shift-right: [w396] -> w316
            shift-left: w308 -> [w397]
            tunnel: w317 -> [w392]
            shift-right: [w390] -> w299
            shift-left: w300 -> [w391]
            tunnel: w284 -> [w348]
            shift-right: [w347] -> w293
            shift-left: w312 -> [w339]
            tunnel: "IB_Clip" -> [w346]
            shift-right: [w336] -> w294
            shift-left: dbl[][] [] ("Y") -> [w337]
            tunnel: ["Full waveform"] -> w298
            i -> [w345]
            stop <- w338 stop-if-true
            w360 = "%[^,],%g,%g,%g,%g,%g,%g," ("format string")
            n98 = Index Array(array=w346, index=w345) -> (element=w344:i32)
            n99 = call "channel_conf_ASIC.vi"("connection ID"=w397, "Ring"=w348, "Clip_sel_b"=w394, "CompBuf_en_b"=TRUE, "error out"=w365, "Att gain"=w395, "Ib_ClipVb"=w344, "Clip_en_b"=FALSE, "Att_en_b"=FALSE) -> ("connection ID out"=w396:refnum<k5>, "error out 2"=w363:errorcluster)  [unwired: 2 in, 3 out]
            n100 = Increment(x=w339) -> (x+1=w347:u16)
            n101 = VISA Write(VISA resource name=w367, write buffer=":CDISPLAY", error in (no error)=w363) -> (VISA resource name out=w369:refnum<visa-resource-name>, error out=w362:errorcluster)  [unwired: 1 out]
            n102 = Multiply(x=0.001, y="y") -> (x*y=w381:dbl)
            n103 = Tick Count (ms)() -> (millisecond timer value=w390:u32)
            n104 = call "Time Delay4"("error in (no error)"=w362, "Delay Time (s)"=w381) -> ("error out"=w380:errorcluster)  [unwired: 9 in]
            n105 = Subtract(x=w390, y=w391) -> (x-y=→"x-y":u32)
            n106 = VISA Write(VISA resource name=w369, write buffer=":MEAS:RES?", error in (no error)=w380) -> (VISA resource name out=w388:refnum<visa-resource-name>, error out=w387:errorcluster)  [unwired: 1 out]
            n107 = VISA Read(VISA resource name=w388, byte count=u32 800, error in (no error)=w387) -> (VISA resource name out=w342:refnum<visa-resource-name>, read buffer=w384:string, error out=w343:errorcluster)  [unwired: 1 out]
            "read buffer 3" <- w384
            n108 = case shown="True" "Full waveform" {
              tunnel: w343 -> [w403 w412]
              tunnel: w342 -> [w402 w414]
              tunnel: [w402 w410] -> w341
              tunnel: [w403 w404] -> w340
              tunnel: w339 -> [_ _]
              tunnel: w337 -> [w401 w407]
              tunnel: [w401 w406] -> w336
              frame #0 {
              }
              frame #1 {
                w413 = i32[] [1, 6] items=["Channel 1"=1, "Channel 2"=2, "Channel 3"=3, "Channel 4"=4, "Function 1"=5, "Function 2"=6, "Function 3"=7, "Function 4"=8, "Memory 1"=9, "Memory 2"=10, "Memory 3"=11, "Memory 4"=12] ("Channels")
                n109 = call-poly <instrlib>:"Read.vi"("error in (no error)"=w412, "Channels"=w413, "VISA resource name"=w414) -> ("error out"=w409:errorcluster, "Waveform Data"=w408:waveform(dbl)[], "VISA resource name out"=w411:refnum<visa-resource-name>)  [unwired: 6 in]
                "Waveform Data" <- w408
                n110 = call "Configure Continuous Acquisition.vi"("error in (no error)"=w409, "VISA resource name"=w411) -> ("error out"=w404:errorcluster, "VISA resource name out"=w410:refnum<visa-resource-name>)  [unwired: 8 in]
                n111 = for {
                  tunnel: w408 -> [w417] mode=indexing
                  tunnel: [w416] -> w405 mode=indexing
                  n112 = Unbundle By Name(w417) -> ("Y"=w416:dbl[], "dt"=→"dt":dbl)
                }
                n113 = Insert Into Array(array=w407, new element=w405) -> (w406:dbl[][])  [unwired: 2 in]
              }
            }
            n114 = Scan From String(format string=w360, input string=w384, error in=w340) -> (remaining string=w377:string, error out=w370:errorcluster, output 5=w359:dbl, output 6=w357:dbl, output 7=w358:dbl)  [unwired: 12 in, 1 out]
            "points quantity" <- w358
            n115 = Scan From String(format string=w360, input string=w377, error in=w370) -> (remaining string=w374:string, error out=w371:errorcluster, output 5=w356:dbl, output 6=w355:dbl)  [unwired: 13 in, 1 out]
            n116 = Scan From String(format string=w360, input string=w374, error in=w371) -> (remaining string=w375:string, error out=w372:errorcluster, output 5=w354:dbl, output 6=w353:dbl)  [unwired: 13 in, 1 out]
            n117 = Scan From String(format string=w360, input string=w375, error in=w372) -> (remaining string=w376:string, error out=w373:errorcluster, output 5=w352:dbl, output 6=w351:dbl)  [unwired: 13 in, 1 out]
            n118 = Scan From String(format string="%[^,],%g,%g,%g,%g,%g,%g", input string=w376, error in=w373) -> (error out=w338:errorcluster, output 5=w350:dbl, output 6=w349:dbl)  [unwired: 13 in, 2 out]
            n119 = Build Array(w359, w357, w356, w355, w354, w353, w352, w351, w350, w349, w358) -> (w379:dbl[])
            "appended array" <- w379
            n120 = Build Array (concatenate)(w400, w348, w395, w344, w394, w379, w392, w339) -> (w399:dbl[])
            n121 = Insert Into Array(array=w398, new element=w399) -> (w378:dbl[][])  [unwired: 2 in]
            "Data output" <- w378
            "bucle" <- w339
          }
          n122 = case shown="True" w298 {
            tunnel: w294 -> [_ w334]
            tunnel: w296 -> [w322 w323]
            tunnel: [w322 w332] -> w297
            tunnel: w295 -> [_ w325]
            tunnel: w293 -> [_ w324]
            frame #0 {
            }
            frame #1 {
              n123 = Number To Decimal String(number=w324) -> (decimal integer string=w331:string)  [unwired: 1 in]
              n124 = Format Into String(initial string="waveform_", w331) -> (resulting string=w329:string)  [unwired: 2 in, 1 out]
              n125 = call "Convert to Dynamic Data"("2D Array"=w334) -> ("Dynamic Data Type"=w333:dynamicdata)  [unwired: 3 in]
              n126 = Concatenate Strings(w329, ".txt" ("string")) -> (w328:string)
              n127 = Build Path(base path=w325, name or relative path=w328) -> (appended path=w326:path)
              n128 = call "Write To Measurement File"("Signals"=w333, "error in (no error)"=w323, "Filename"=w326) -> ("error out"=w332:errorcluster)  [unwired: 14 in, 2 out]
            }
          }
        }
      }
      n129 = TCP Close Connection(connection ID=w103, error in (no error)=w104) -> (error out=w105:errorcluster)  [unwired: 1 in, 1 out]
      n130 = stacked-sequence {
        tunnel: w105 -> [w193 _]
        tunnel: [w192 _] -> w125
        tunnel: w116 -> [w191 _]
        tunnel: [w190 _] -> w96
        frame #0 {
          w194 = u16 1 items=["Immediate", "Internal", "External", "Software Trigger Function"] ("Trigger Source (0: Immediate)")
          w195 = u16 0 items=["Edge", "Level"] ("Trigger Mode (0: Edge)")
          n131 = call <instrlib>:"Configure Trigger.vi"("Trigger Source (0: Immediate)"=w194, "error in (no error)"=w193, "Trigger Mode (0: Edge)"=w195, "VISA resource name"=w191) -> ("error out"=w192:errorcluster, "VISA resource name out"=w190:refnum<visa-resource-name>)  [unwired: 6 in]
        }
        frame #1 {
          n132 = local write "End 2"(TRUE ("End 2")) -> ()
        }
      }
      n133 = Unbundle By Name(w94) -> ("report out"=w121:refnum<class "NI_report.lvclass">)
      n134 = Number To Engineering String(4:w124) -> (0:w122:string[][])  [unwired: 3 in]
      n135 = call "AddTableReport.vi"("Table title"="Check calibration precision", "Report Enable"="Report Enable", "Data"=w122, "error in"=w125, "report in"=w121) -> ("error out"=w119:errorcluster, "report out"=w126:refnum<class "NI_report.lvclass">)  [unwired: 5 in]
      n136 = Bundle By Name(cluster=w94, "report out"=w126, "AWG VISA"=w96, "Oscilloscope  VISA"=w95) -> (w117:T1)
    }
  }
  "Instrument VISA out" <- w14
  n137 = Unbundle By Name(w14) -> ("AWG VISA"=w17:refnum<visa-resource-name>, "Oscilloscope  VISA"=w18:refnum<visa-resource-name>)
  n138 = call <instrlib>:"Close.vi"("error in (no error)"=w16, "VISA resource name"=w18) -> ("error out"=w19:errorcluster)  [unwired: 9 in]
  n139 = call <instrlib>:"Close.vi"("error in (no error)"=w19, "VISA resource name"=w17) -> ("error out"=→"error out":errorcluster)  [unwired: 9 in]
